vi "Msg.vi"(7 "Actor in":refnum<class "Actor.lvclass">, 11 "Msg in":refnum<class "Msg.lvclass">) -> (5 "Actor out":refnum<class "Actor.lvclass">)   [LabVIEW 2021, in "jettl.lvlib" / "Msg.lvclass"]
uses:
  Msg.lvclass
  Actor/Actor.lvclass
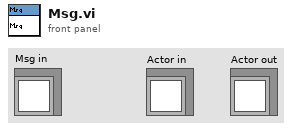
[diagram p1: front panel]
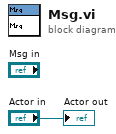
[diagram p0: block diagram]
diagram:
  "Actor out" <- "Actor in"
